vi "Echo_Disabled.vi"() -> ()   [LabVIEW 2012]
uses:
  <vilib>/Rock Robotics/WPI/Joystick/WPI_JoystickDeviceEnum.ctl
  <vilib>/Rock Robotics/WPI/DriverStation/DriverStationLCD/WPI_DriverStationLCDLCDLine.ctl
panel:
  in  "Numeric":i32
  # "This VI helps you select autonomous modes.\nEnter file path arrays for your autonomous\nin the block diagram under a number, and\nchange the constant to true.\n\nThe VI allows you to scroll through the modes\nby using buttons on your joystick.  The default\njoystick is in USB 1 and the default buttons for\nscrolling are 1 and 2.  This is easily altered by \nlooking at the block diagram."
  # "You must place this VI in Disabled, without any inputs,\nand outside any while loops except for the main while\nloop containing Disabled.vi"
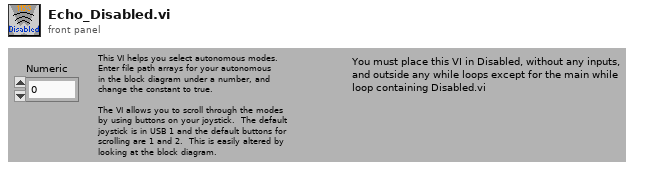
[diagram p1: front panel]
types:
  T1 = typedef "WPI_JoystickDeviceEnum.ctl" = enum16{"USB 1", "USB 2", "USB 3", "USB 4", "Kinect 1", "Kinect 2"}
  T2 = typedef "WPI_JoystickDevRef.ctl" = cluster{"Device":T1}
  T3 = typedef "WPI_JoystickButtonState.ctl" = cluster{"Button 1":bool, "Button 2":bool, "Button 3":bool, "Button 4":bool, "Button 5":bool, "Button 6":bool, "Button 7":bool, "Button 8":bool, "Button 9":bool, "Button 10":bool, "Button 11":bool, "Button 12":bool}
  T4 = typedef "WPI_DriverStationLCDLCDLine.ctl" = enum16{"Main - Line 1", "User - Line 2", "User - Line 3", "User - Line 4", "User - Line 5", "User - Line 6"}
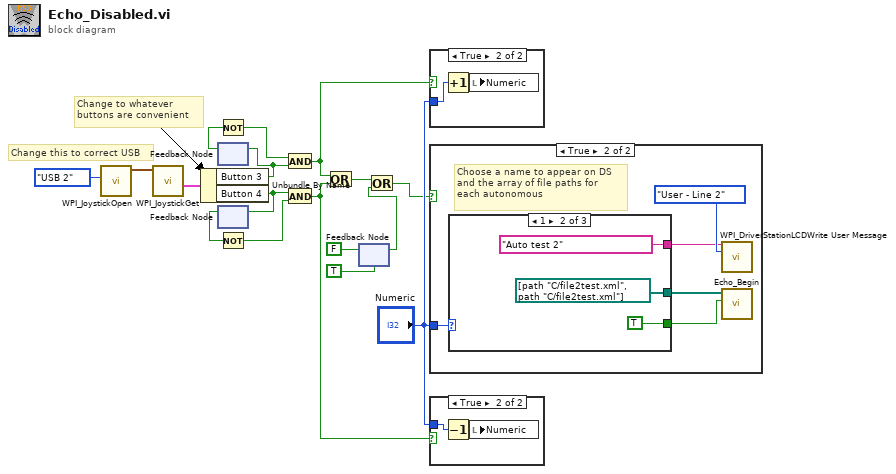
[diagram p0: block diagram]
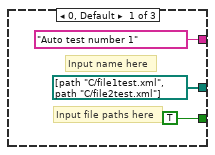
[diagram p3: hidden frame]
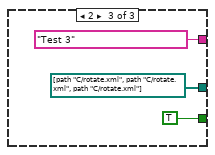
[diagram p4: hidden frame]
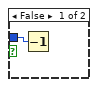
[diagram p5: hidden frame]
diagram:
  # "Change to whatever\nbuttons are convenient"
  # "Change this to correct USB"
  n1 = call <vilib>:"WPI_JoystickOpen.vi"("JoystickDevice"=WPI_JoystickDeviceEnum."USB 2") -> ("JoystickDevRef"=w17:T2)  [unwired: 10 out]
  n2 = call <vilib>:"WPI_JoystickGet.vi"("JoystickDevRef"=w17) -> ("Buttons"=w15:T3)  [unwired: 1 in, 5 out]
  n3 = Unbundle By Name(w15) -> ("Button 3"=w1:bool, "Button 4"=w3:bool)
  n4 = feedback-in #1(w1) -> ()
  n5 = feedback #1() -> (w12:bool)  [unwired: 1 out]
  n6 = Not(x=w12) -> (.not. x?=w13:bool)
  n7 = feedback-in #2(w3) -> ()
  n8 = feedback #2() -> (w11:bool)  [unwired: 1 out]
  n9 = Not(x=w11) -> (.not. x?=w2:bool)
  n10 = And(x=w13, y=w1) -> (x .and. y?=w9:bool)
  n11 = And(x=w3, y=w2) -> (x .and. y?=w8:bool)
  n12 = Or(x=w9, y=w8) -> (x .or. y?=w10:bool)
  n13 = feedback-in #3(FALSE) -> ()
  n14 = feedback #3(TRUE) -> (w5:bool)
  n15 = Or(x=w10, y=w5) -> (x .or. y?=w7:bool)
  n16 = case shown="True" w9 {
    tunnel: "Numeric" -> [_ w19]
    frame False {
    }
    frame True {
      n17 = Increment(x=w19) -> (x+1=w18:i32)
      n18 = local write "Numeric"(w18) -> ()
    }
  }
  n19 = case shown="True" w7 {
    tunnel: "Numeric" -> [_ w22]
    frame False {
    }
    frame True {
      # "Choose a name to appear on DS\nand the array of file paths for\neach autonomous"
      n20 = case shown="1" w22 {
        tunnel: ["Auto test number 1" "Auto test 2" "Test 3"] -> w23
        tunnel: [path[] [path "C:/file1test.xml", path "C:/file2test.xml"] path[] [path "C:/file2test.xml", path "C:/file2test.xml"] path[] [path "C:/rotate.xml", path "C:/rotate.xml", path "C:/rotate.xml"]] -> w21
        tunnel: [TRUE TRUE TRUE] -> w20
        frame 0, Default {
          # "Input file paths here"
          # "Input name here"
        }
        frame 1 {
        }
        frame 2 {
        }
      }
      n21 = call <vilib>:"WPI_DriverStationLCDWrite User Message.vi"("line text"=w23, "line"=WPI_DriverStationLCDLCDLine."User - Line 2") -> ()  [unwired: 3 in, 11 out]
      n22 = call "Echo_Begin.vi"("Read"=w20, "Files"=w21) -> ()  [unwired: 10 out]
    }
  }
  n23 = case shown="True" w8 {
    tunnel: "Numeric" -> [w34 w36]
    frame False {
      n24 = Decrement(x=w34) -> ()  [unwired: 1 out]
    }
    frame True {
      n25 = Decrement(x=w36) -> (x-1=w35:i32)
      n26 = local write "Numeric"(w35) -> ()
    }
  }
